vi "Verify.vi"(8 "error in (no error)":errorcluster, 9 "Value":string, 10 "Key":string, 11 "LUT in":refnum<class "LUT.lvclass">) -> (0 "error out":errorcluster, 2 "Verified?":bool, 3 "LUT out":refnum<class "LUT.lvclass">)   [LabVIEW 2016, in "LUT.lvclass"]
uses:
  LUT.lvclass
  LUT.lvclass/LUT.ctl
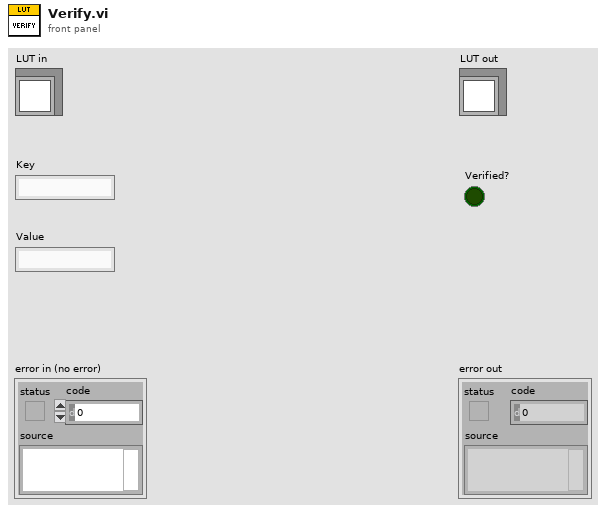
[diagram p1: front panel]
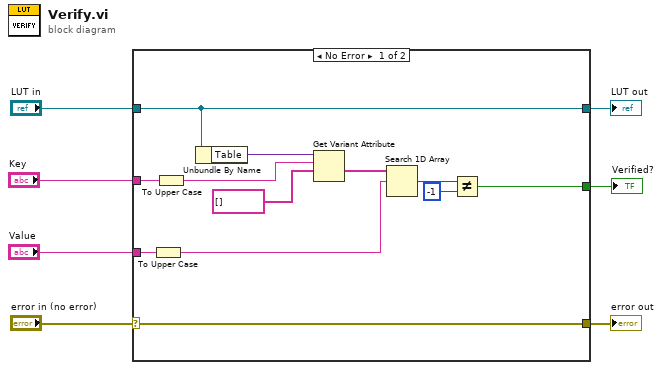
[diagram p0: block diagram]
diagram:
  n1 = case shown="No Error" "error in (no error)" {
    selector: "error in (no error)" -> [w19 w21]
    tunnel: [w19 w21] -> w6
    tunnel: [w18 w20] -> w4
    tunnel: "LUT in" -> [w18 w20]
    tunnel: "Key" -> [w16 _]
    tunnel: "Value" -> [w13 _]
    tunnel: [w8 _] -> w1
    frame No Error {
      n2 = To Upper Case(1:w13) -> (0:w11:string)
      n3 = To Upper Case(1:w16) -> (0:w12:string)
      n4 = Unbundle By Name(w18) -> ("Table"=w17:variant)
      n5 = Get Variant Attribute(Variant=w17, name=w12, default value (empty Variant)=string[] []) -> (value=w14:string[])  [unwired: 1 in, 3 out]
      n6 = Search 1D Array(1D array=w14, element=w11) -> (index of element=w10:i32)  [unwired: 1 in]
      n7 = Not Equal?(x=w10, y=-1) -> (x != y?=w8:bool)
    }
    frame Error {
    }
  }
  "error out" <- w6
  "LUT out" <- w4
  "Verified?" <- w1
